vi "serialLabView.vi"() -> ()   [LabVIEW 2017]
doc: "This example performs writes and reads on a serial port, as directed by the user. You can press the Write and Read buttons, and change the Read Count, while the example is running.\n\nThe parameters set for the serial port must match the parameters of the connected instrument or device. In this example, the Read Count parameter specifies the number of bytes that the serial port reads. If there were more bytes at the port than the specified number, those bytes would not be read. If there were less bytes at the port than the specified number, you would receive a timeout error.\n\nThis example expands upon the flow control options for XON and XOFF, allowing the user to choose those control characters. Also, the user can enable or disable a termination character. Some devices require a termination character in order to identify the end of command strings. Some devices send a termination character to signify the end of data to be read. This example shows how you can end the Read operation once a termination character is detected in the buffer and/or append a termination character at the end of the Write data."
uses:
  Program Files/National Instruments/LabVIEW 2017/examples/Instrument IO/Serial/support/Serial - Settings.ctl
  Program Files/National Instruments/LabVIEW 2017/examples/Instrument IO/Serial/support/Serial - XON-XOFF Characters.ctl
  Program Files/National Instruments/LabVIEW 2017/examples/Instrument IO/Serial/support/Serial - ASCII Characters.ctl
  <vilib>/Math Plots/2D Math Plots/XY Plot Matrix/XY Plot Matrix XCtrl/XY Plot Matrix.xctl
  <vilib>/Instr/_visa.llb/VISA Configure Serial Port (Instr).vi
  <vilib>/Math Plots/2D Math Plots/XY Plot Matrix/XY Plot Matrix Datatype/XY Plot Matrix Datatype.lvclass
panel:
  out "XY Plot Matrix":refnum<class "XY Plot Matrix Datatype.lvclass">[](xcontrol)
  in  "Termination Character":u8=10 format="%.0x"
  in  "End Write on Termination Character?":bool=TRUE
  in  "Stop":bool
  in  "Command":string="*IDN?"
  in  "Read Count":u32=1000
  out "Response":string
  in  "Write":bool
  in  "Read":bool
  in  "XON/XOFF Characters":T1={"XON"=enum."DC1", "XOFF"=enum."DC3"}
  in  "Serial Settings":T3={"baud rate"=9600, "data bits"=8, "parity"=enum."None", "stop bits"=10, "flow control"=0} {"flow control" items=["None"=0, "XON/XOFF"=1, "RTS/CTS"=2, "DTR/DSR"=4]; "stop bits" items=["1.0"=10, "1.5"=15, "2.0"=20]; "data bits" min=5 max=8 step=1; "baud rate" items=["75"=75, "110"=110, "134"=134, "150"=150, "300"=300, "600"=600, "1200"=1200, "1800"=1800, "2400"=2400, "4800"=4800, "7200"=7200, "9600"=9600, "14400"=14400, "19200"=19200, "28800"=28800, "38400"=38400, "56000"=56000, "57600"=57600, "115200"=115200, "128000"=128000, "230400"=230400]}
  in  "End Read on Termination Character?":bool=TRUE
  in  "VISA resource name":refnum<visa-resource-name>="COM1"
  # "Overview: Demonstrates the use of the VISA functions to write commands to and read responses from a serial instrument continuously in a loop.\nRequirements: NI-VISA Driver\nInstructions:\n1. Run the VI.\n2. Specify a Command and click the Write button.\n3. Read a Response by clicking the Read button.\n4. Click Stop to stop the VI."
  # "0xA is equivalent to a '\\n' character, which is a line feed."
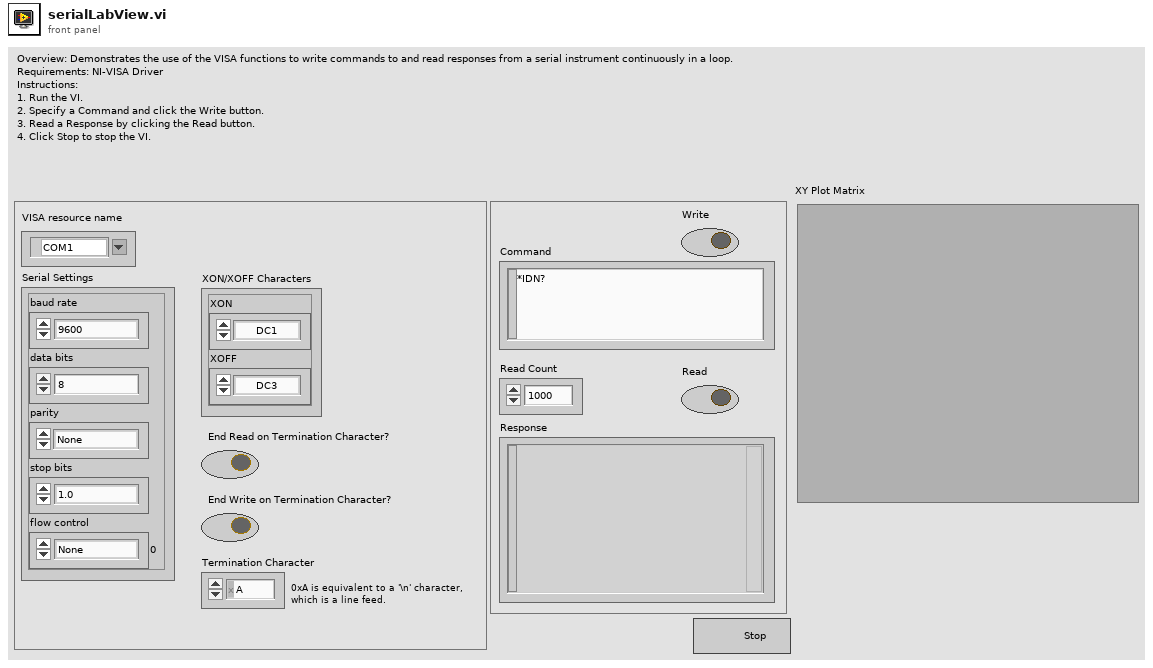
[diagram p1: front panel]
types:
  T1 = typedef "Serial - XON-XOFF Characters.ctl" = cluster{"XON":T2, "XOFF":T2}
  T2 = typedef "Serial - ASCII Characters.ctl" = enum16{"NUL", "SOH", "STX", "ETX", "EOT", "ENQ", "ACK", "BEL", "BS", "HT", "LF", "VT", "FF", "CR", "SO", "SI", "DLE", "DC1", "DC2", "DC3", "DC4", "NAK", "SYN", "ETB", "CAN", "EM", "SUB", "ESC", "FS", "GS", "RS", "US", "SP", "!", "\"", "#", "$", "%", "&", "'", "(", ")", "*", "+", ",", "- (-)", ".", "/", "0", "1", "2", "3", "4", "5", "6", "7", "8", "9", ":", ";", "<", "=", ">", "?", "@", "A", "B", "C", "D", "E", "F", "G", "H", "I", "J", "K", "L", "M", "N", "O", "P", "Q", "R", "S", "T", "U", "V", "W", "X", "Y", "Z", "[", "\\", "]", "^", "_", "`", "a", "b", "c", "d", "e", "f", "g", "h", "i", "j", "k", "l", "m", "n", "o", "p", "q", "r", "s", "t", "u", "v", "w", "x", "y", "z", "{", "|", "}", "~"}
  T3 = typedef "Serial - Settings.ctl" = cluster{"baud rate":u32, "data bits":u16, "parity":enum16{"None", "Odd", "Even", "Mark", "Space"}, "stop bits":u16, "flow control":u16}
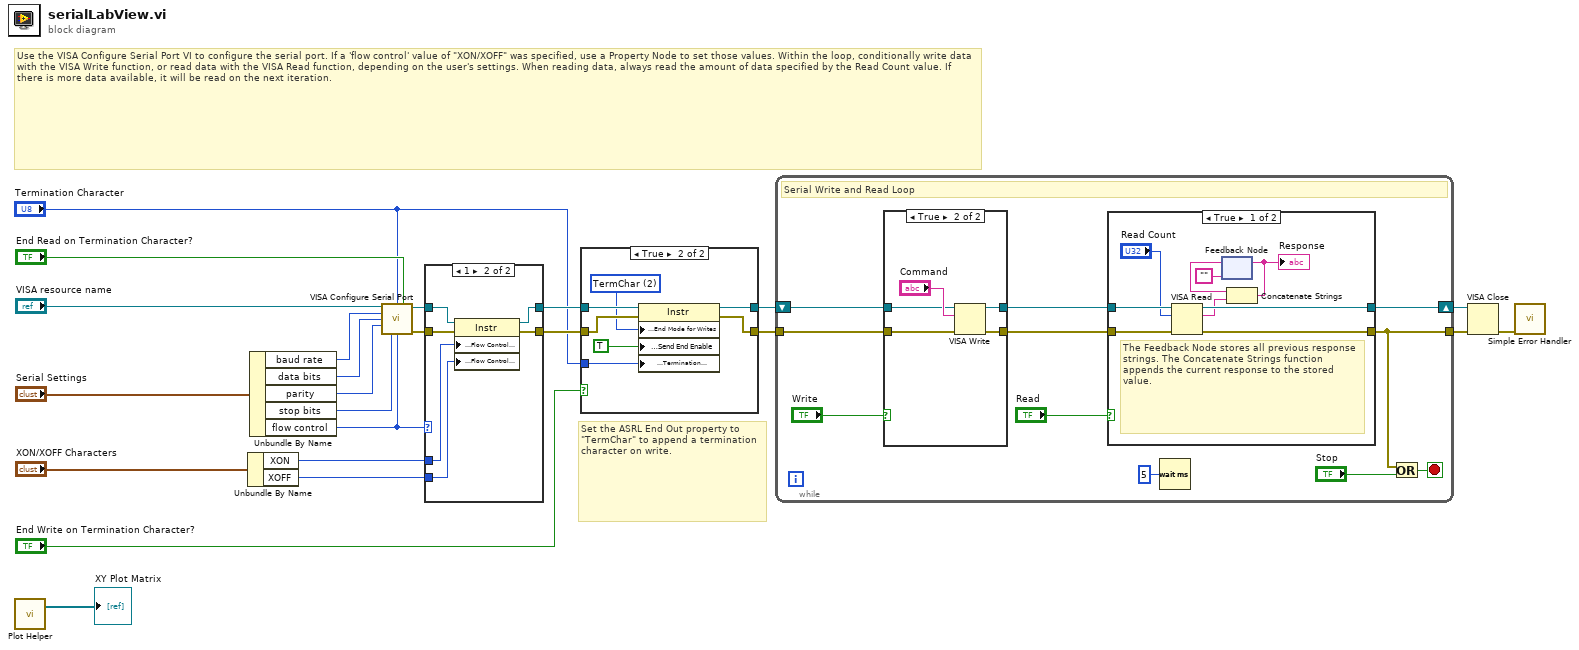
[diagram p0: block diagram]
diagram:
  # "Set the ASRL End Out property to \"TermChar\" to append a termination character on write."
  # "Use the VISA Configure Serial Port VI to configure the serial port. If a 'flow control' value of \"XON/XOFF\" was specified, use a Property Node to set those values. Within the loop, conditionally write data with the VISA Write function, or read data with the VISA Read function, depending on the user's settings. When reading data, always read the amount of data specified by the Read Count value. If there is more data available, it will be read on the next iteration."
  n1 = call <vilib>:"Plot Helper.vi"() -> ("2D Plotmatrix Class Obj Array out"=→"XY Plot Matrix":refnum<class "XY Plot Matrix Datatype.lvclass">[])  [unwired: 4 in, 7 out]
  n2 = Unbundle By Name("XON/XOFF Characters") -> ("XON"=w9:T2, "XOFF"=w8:T2)
  n3 = Unbundle By Name("Serial Settings") -> ("baud rate"=w16:u32, "data bits"=w17:u16, "parity"=w18:enum16{"None", "Odd", "Even", "Mark", "Space"}, "stop bits"=w19:u16, "flow control"=w10:u16)
  n4 = call-poly "VISA Configure Serial Port"("VISA resource name"="VISA resource name", "termination char\n(0xA = '\\n' = LF)"="Termination Character", "Enable Termination\nChar (T)"="End Read on Termination Character?", "baud rate (9600)"=w16, "data bits (8)"=w17, "parity (0:none)"=w18, "stop bits (10: 1 bit)"=w19, "flow control (0:none)"=w10) -> ("VISA resource name out"=w20:refnum<visa-resource-name>, "error out"=w21:errorcluster)  [unwired: 2 in, 4 out]
  n5 = case shown="1" w10 {
    tunnel: [w24 w31] -> w7
    tunnel: [w25 w30] -> w5
    tunnel: w21 -> [w24 w29]
    tunnel: w20 -> [w25 w28]
    tunnel: w9 -> [_ w27]
    tunnel: w8 -> [_ w26]
    frame Default {
    }
    frame 1 {
      n6 = property class="Instr"(reference=w28, error in=w29, "Serial Settings:Flow Control XON Character"=w27, "Serial Settings:Flow Control XOFF Character"=w26) -> (reference out=w30:refnum<visa-resource-name>, error out=w31:errorcluster)
    }
  }
  n7 = case shown="True" "End Write on Termination Character?" {
    tunnel: w5 -> [w32 w40]
    tunnel: w7 -> [w33 w39]
    tunnel: [w32 w38] -> w4
    tunnel: [w33 w37] -> w6
    tunnel: "Termination Character" -> [_ w35]
    frame False {
    }
    frame True {
      w36 = u16 2 items=["None", "LastBit", "TermChar", "Break"] ("Serial Settings:Serial End Mode for Writes")
      n8 = property class="Instr"(reference=w40, error in=w39, "Serial Settings:End Mode for Writes"=w36, "Message Based Settings:Send End Enable"=TRUE, "Message Based Settings:Termination Character"=w35) -> (reference out=w38:refnum<visa-resource-name>, error out=w37:errorcluster)
    }
  }
  n9 = while {
    shift-right: [w51] -> w11
    shift-left: w4 -> [w50]
    tunnel: w6 -> [w49]
    tunnel: [w43] -> w12
    stop <- w44 stop-if-true
    # "Serial Write and Read Loop"
    n10 = case shown="True" "Write" {
      tunnel: w50 -> [w53 w57]
      tunnel: w49 -> [w52 w56]
      tunnel: [w53 w55] -> w48
      tunnel: [w52 w54] -> w47
      frame False {
      }
      frame True {
        n11 = VISA Write(VISA resource name=w57, write buffer="Command", error in (no error)=w56) -> (VISA resource name out=w55:refnum<visa-resource-name>, error out=w54:errorcluster)  [unwired: 1 out]
      }
    }
    n12 = case shown="True" "Read" {
      tunnel: [w65 w69] -> w51
      tunnel: w48 -> [w67 w69]
      tunnel: [w63 w68] -> w43
      tunnel: w47 -> [w66 w68]
      frame True {
        # "The Feedback Node stores all previous response strings. The Concatenate Strings function appends the current response to the stored value."
        n13 = VISA Read(VISA resource name=w67, byte count="Read Count", error in (no error)=w66) -> (VISA resource name out=w65:refnum<visa-resource-name>, read buffer=w62:string, error out=w63:errorcluster)  [unwired: 1 out]
        n14 = feedback #1("") -> (w61:string)
        n15 = Concatenate Strings(w61, w62) -> (w60:string)
        "Response" <- w60
        n16 = feedback-in #1(w60) -> ()
      }
      frame False {
      }
    }
    n17 = Wait (ms)(milliseconds to wait=u32 5) -> ()  [unwired: 1 out]
    n18 = Or(x=w43, y="Stop") -> (x .or. y?=w44:bool)
  }
  n19 = VISA Close(VISA resource name=w11, error in (no error)=w12) -> (error out=w13:errorcluster)
  n20 = call <vilib>:"Simple Error Handler.vi"("error in (no error)"=w13) -> ()  [unwired: 1 in, 8 out]
